vi "connection_process.vi"(6 "timeout (ms)":i32=1000, 11 "Connection":refnum<class "Connection.lvclass">) -> ()   [LabVIEW 2013, in "MQTT_Connection.lvlib" / "Connection.lvclass"]
uses:
  Connection.lvclass
  Connection.lvclass/Connection.ctl
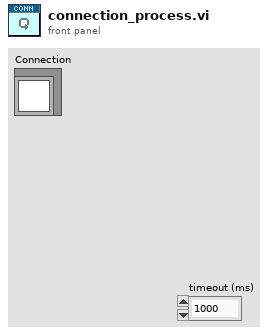
[diagram p1: front panel]
types:
  T1 = cluster{"Connection out":refnum<class "Connection.lvclass">, "error out":errorcluster}
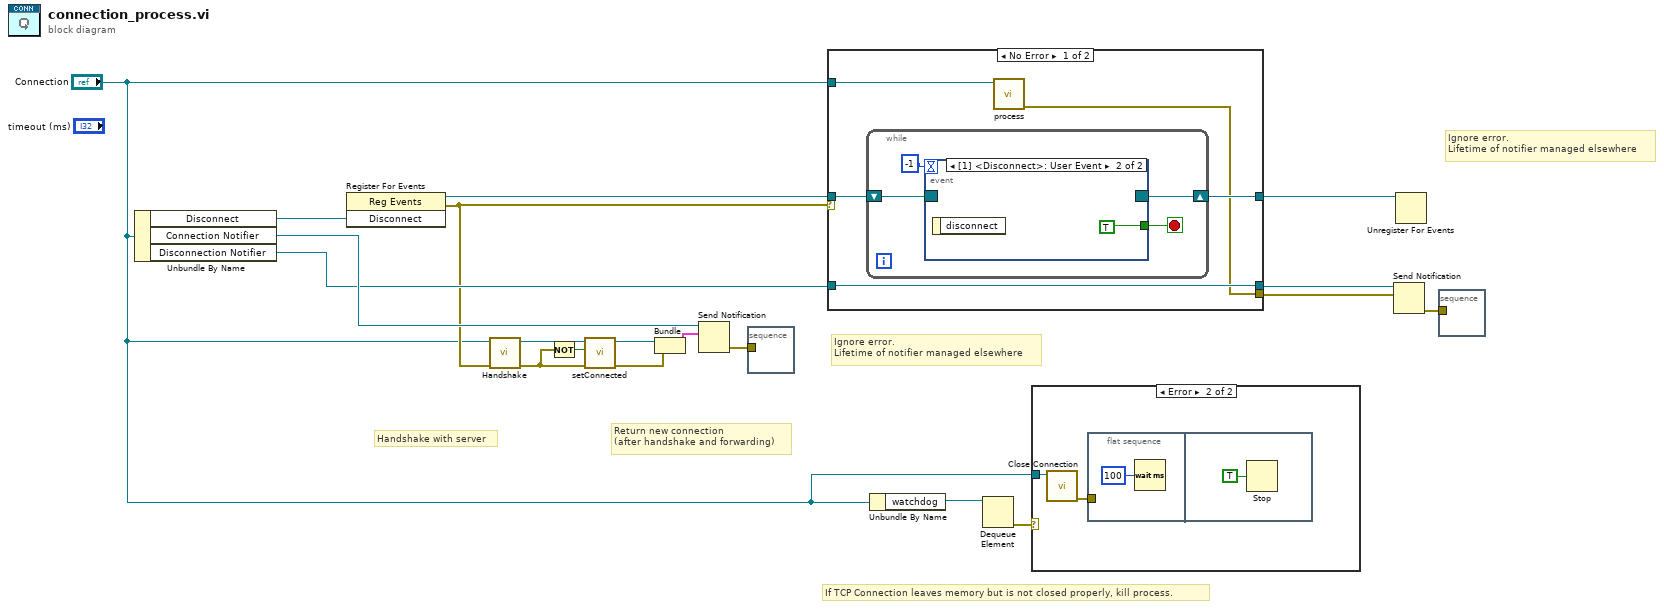
[diagram p0: block diagram]
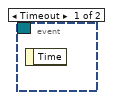
[diagram p3: hidden frame]
diagram:
  # "Return new connection\n(after handshake and forwarding)"
  # "Handshake with server"
  # "If TCP Connection leaves memory but is not closed properly, kill process."
  # "Ignore error.\nLifetime of notifier managed elsewhere"
  # "Ignore error.\nLifetime of notifier managed elsewhere"
  n1 = Unbundle By Name("Connection") -> ("Disconnect"=w16:refnum<user-event>, "Connection Notifier"=w15:refnum<notifier>, "Disconnection Notifier"=w12:refnum<notifier>)
  n2 = register-events(w16) -> (reference out=w17:refnum<event-registration>, error out=w9:errorcluster)  [unwired: 2 in]
  n3 = call-dynamic "Handshake.vi"("error in (no error)"=w9, "Connection in"="Connection") -> ("error out"=w1:errorcluster, "Connection out"=w4:refnum<class "Connection.lvclass">)  [unwired: 8 in]
  n4 = Not(x=w1) -> (.not. x?=w2:bool)
  n5 = call "setConnected.vi"("error in (no error)"=w1, "connected"=w2, "Connection in"=w4) -> ("error out"=w5:errorcluster, "Connection out"=w3:refnum<class "Connection.lvclass">)  [unwired: 7 in]
  n6 = Bundle("Connection out"=w3, "error out"=w5) -> (w19:T1)  [unwired: 1 in]
  n7 = Send Notification(notification=w19, notifier=w15) -> (error out=w7:errorcluster)  [unwired: 1 in, 1 out]
  n8 = stacked-sequence {
    tunnel: w7 -> [_]
    frame #0 {
    }
  }
  n9 = case shown="No Error" w9 {
    selector: w9 -> [_ w31]
    tunnel: [w24 w32] -> w18
    tunnel: w17 -> [w23 w32]
    tunnel: [w20 w31] -> w14
    tunnel: w12 -> [w22 w30]
    tunnel: [w22 w30] -> w13
    tunnel: "Connection" -> [w21 _]
    frame No Error {
      n10 = while {
        shift-right: [w27] -> w24
        shift-left: w23 -> [w26]
        stop <- w25 stop-if-true
        n11 = event shown="[1] <Disconnect>: User Event" {
          selector: w26 -> [_ _]
          dyn-events: [_ _] -> w27
          timeout: -1 -> [_ _]
          tunnel: [_ TRUE] -> w25
          event Timeout {
            n12 = event-data() -> ()  [unwired: 1 in, 1 out]
          }
          event User Event {
            n13 = event-data() -> ()  [unwired: 1 in, 1 out]
          }
        }
      }
      n14 = call-dynamic "process.vi"("Connection in"=w21) -> ("error out"=w20:errorcluster)  [unwired: 9 in, 1 out]
    }
    frame Error {
    }
  }
  n15 = Unbundle By Name("Connection") -> ("watchdog"=w11:refnum<queue>)
  n16 = Dequeue Element(queue=w11) -> (error out=w10:errorcluster)  [unwired: 2 in, 3 out]
  n17 = case shown="Error" w10 {
    tunnel: "Connection" -> [_ w34]
    frame No Error {
    }
    frame Error {
      n18 = call "Close Connection.vi"("Connection in"=w34) -> ("error out"=w33:errorcluster)  [unwired: 9 in, 1 out]
      n19 = flat-sequence {
        tunnel: w33 -> [_]
        frame #0 {
          n20 = Wait (ms)(milliseconds to wait=u32 100) -> ()  [unwired: 1 out]
        }
        frame #1 {
          n21 = Stop(stop? (T)=TRUE) -> ()
        }
      }
    }
  }
  n22 = Send Notification(notification=w14, notifier=w13) -> (error out=w6:errorcluster)  [unwired: 1 in, 1 out]
  n23 = Unregister For Events(event registration refnum=w18) -> ()  [unwired: 1 in, 1 out]
  n24 = stacked-sequence {
    tunnel: w6 -> [_]
    frame #0 {
    }
  }
